vi "Theta 5.vi"(7 "XYZ_6":dbl[](array[numeric])=[0.0, 0.0, 0.0], 10 "theta_4":dbl, 11 "6R Type 3 Serial Arm Class in":refnum<class "NI_Robotics_6R Type 3 Serial Arm Class.lvclass">) -> (1 "valid?":bool, 2 "theta_5":dbl, 3 "6R Type 3 Serial Arm Class out":refnum<class "NI_Robotics_6R Type 3 Serial Arm Class.lvclass">)   [LabVIEW 2017, in "NI_Robotics_6R Type 3 Serial Arm Class.lvclass"]
uses:
  <vilib>/robotics/Kinematics/Analytical/6R/Type 3/NI_Robotics_6R Type 3 Serial Arm Class.lvclass
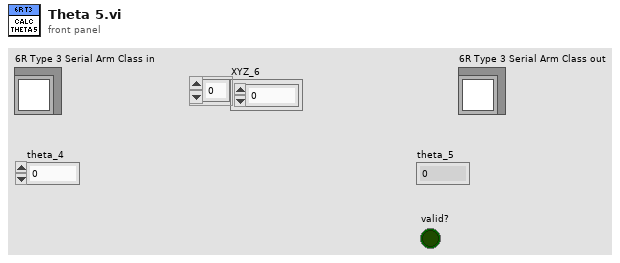
[diagram p1: front panel]
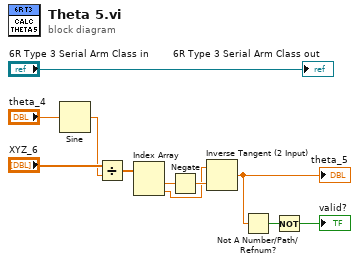
[diagram p0: block diagram]
diagram:
  n1 = Sine(x="theta_4") -> (sin(x)=w8:dbl)
  n2 = Divide(x="XYZ_6", y=w8) -> (x/y=w7:dbl[])
  n3 = Index Array(array=w7) -> (element #1=w6:dbl, element #2=w4:dbl)  [unwired: 2 in]
  n4 = Negate(x=w6) -> (-x=w5:dbl)
  n5 = Inverse Tangent (2 Input)(1:w5, 2:w4) -> (0:w1:dbl)
  "theta_5" <- w1
  n6 = Not A Number/Path/Refnum?(number/path/refnum=w1) -> (NaN/Path/Refnum?=w2:bool)
  n7 = Not(x=w2) -> (.not. x?=→"valid?":bool)
  "6R Type 3 Serial Arm Class out" <- "6R Type 3 Serial Arm Class in"
